vi "Read T Controller Settings.vi"(8 "error in (no error)":errorcluster, 11 "Neocera LTC-21 in":refnum<class "Neocera LTC-21.lvclass">) -> (0 "error out":errorcluster, 1 "Heater level":dbl, 2 "Heater mode":T1(ring), 3 "Neocera LTC-21 out":refnum<class "Neocera LTC-21.lvclass">, 4 "PID":cluster{"P":dbl, "I":dbl, "D":dbl}, 5 "Hater range":dbl, 7 "Set point":dbl)   [LabVIEW 2015, in "Neocera LTC-21.lvclass"]
uses:
  Neocera LTC-21.lvclass
  Instrument/Instrument.lvclass
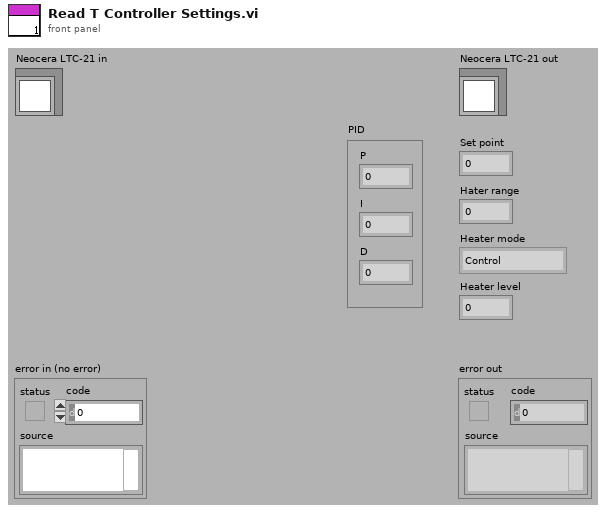
[diagram p1: front panel]
types:
  T1 = enum16{"Control", "Monitor", "Manual Heat", "Controller is in OFF mode", "Autotune is in progress"}
  T2 = enum16{"Control", "Monitor", "Manual Heat", "Controller is in OFF mode", "Autotune is in progress"}[]
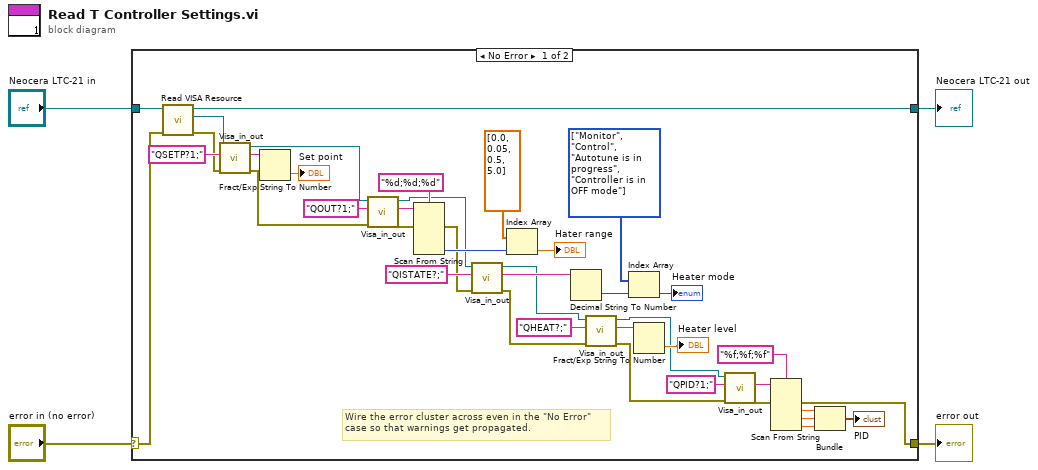
[diagram p0: block diagram]
diagram:
  n1 = case shown="No Error" "error in (no error)" {
    selector: "error in (no error)" -> [w42 w46]
    tunnel: [w10 w46] -> w3
    tunnel: [w43 w45] -> w1
    tunnel: "Neocera LTC-21 in" -> [w44 w45]
    frame No Error {
      w36 = T2 [enum."Monitor", enum."Control", enum."Autotune is in progress", enum."Controller is in OFF mode"] items=["Control", "Monitor", "Manual Heat", "Controller is in OFF mode", "Autotune is in progress"]
      # "Wire the error cluster across even in the \"No Error\"\ncase so that warnings get propagated."
      n2 = call "Read VISA Resource.vi"("error in (no error)"=w42, "Instrument.lvclass in"=w44) -> ("error out"=w16:errorcluster, "VISA Resource"=w20:refnum<visa-resource-name>, "Instrument.lvclass out"=w43:refnum<class "Neocera LTC-21.lvclass">)  [unwired: 7 out]
      n3 = call "Visa_in_out.vi"("error in (no error)"=w16, "write buffer"="QSETP?1;", "VISA resource name"=w20) -> ("error out"=w17:errorcluster, "read buffer"=w21:string, "VISA resource name out"=w19:refnum<visa-resource-name>)  [unwired: 1 in, 5 out]
      n4 = Fract/Exp String To Number(string=w21) -> (number=→"Set point":dbl)  [unwired: 4 out]
      n5 = call "Visa_in_out.vi"("error in (no error)"=w17, "write buffer"="QOUT?1;", "VISA resource name"=w19) -> ("error out"=w25:errorcluster, "read buffer"=w29:string, "VISA resource name out"=w23:refnum<visa-resource-name>)  [unwired: 1 in, 5 out]
      n6 = Scan From String(format string="%d;%d;%d", input string=w29, error in=w25) -> (error out=w24:errorcluster, output 3=w27:i32)  [unwired: 6 in, 2 out]
      n7 = call "Visa_in_out.vi"("error in (no error)"=w24, "write buffer"="QISTATE?;", "VISA resource name"=w23) -> ("error out"=w32:errorcluster, "read buffer"=w37:string, "VISA resource name out"=w33:refnum<visa-resource-name>)  [unwired: 1 in, 5 out]
      n8 = Index Array(array=dbl[] [0.0, 0.05, 0.5, 5.0], index=w27) -> (element=→"Hater range":dbl)
      n9 = Decimal String To Number(string=w37) -> (number=w35:i32)  [unwired: 2 in, 1 out]
      n10 = call "Visa_in_out.vi"("error in (no error)"=w32, "write buffer"="QHEAT?;", "VISA resource name"=w33) -> ("error out"=w13:errorcluster, "read buffer"=w40:string, "VISA resource name out"=w5:refnum<visa-resource-name>)  [unwired: 1 in, 5 out]
      n11 = Index Array(array=w36, index=w35) -> (element=→"Heater mode":T1)
      n12 = Fract/Exp String To Number(string=w40) -> (number=→"Heater level":dbl)  [unwired: 4 out]
      n13 = call "Visa_in_out.vi"("error in (no error)"=w13, "write buffer"="QPID?1;", "VISA resource name"=w5) -> ("error out"=w11:errorcluster, "read buffer"=w14:string)  [unwired: 1 in, 6 out]
      n14 = Scan From String(format string="%f;%f;%f", input string=w14, error in=w11) -> (error out=w10:errorcluster, output 1=w9:dbl, output 2=w8:dbl, output 3=w7:dbl)  [unwired: 4 in, 2 out]
      n15 = Bundle(w9, w8, w7) -> (→"PID":cluster{dbl, dbl, dbl})  [unwired: 1 in]
    }
    frame Error {
    }
  }
  "error out" <- w3
  "Neocera LTC-21 out" <- w1
